vi "flash_RPCV3.vi"() -> ()   [LabVIEW 2017]
panel:
  in  "UDP Update":bool=TRUE
  out "error out 2":errorcluster
  out "Out 2":u8=2 format="%.0x"
  in  "Firmware":u16(ring)=2 items=["TDC"=4, "Middle"=3, "Backend"=2]
  out "Out":u8=1 format="%.0x"
  out "字符串 2":string
  out "concatenated string":string
  in  "Register_Base_Address":u32=512 format="%x"
  in  "start":bool=TRUE
  out "Current IP address":string="10.3.173.20"
  in  "IP address list":string[](array[string])=["10.3.173.20"]
  in  "回读":bool
  out "Current Progress":u32(slide)=6712320 scale=0.0..6712112.0
  out "error out":errorcluster={"status"=TRUE, "code"=1, "source"="TCP Close Connection in flash_RPCV3.vi"}
  out "appended array":bool[](array[boolean])
  out "Process":u32=6712320
  in  "error in (no error)":errorcluster
  in  "Read (TRUE)":bool
  out "byte data":string
  out "Total size (in bytes)":i64=6712112
  in  "bin file path (use dialog)":path=path "G:/rpc/aggregate/WR/firmware/NEM_DEVB/project_1.runs/impl_1/top.bin"
  # "FF80 0001 0000 0209 13"
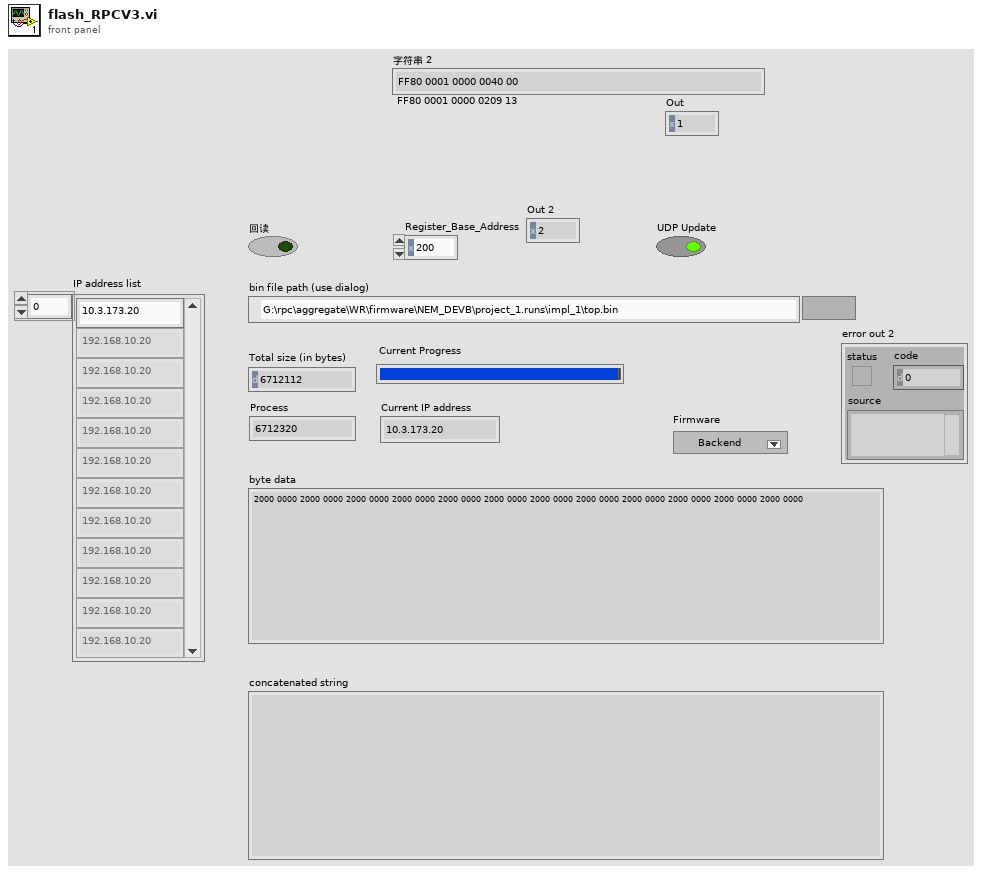
[diagram p1: front panel]
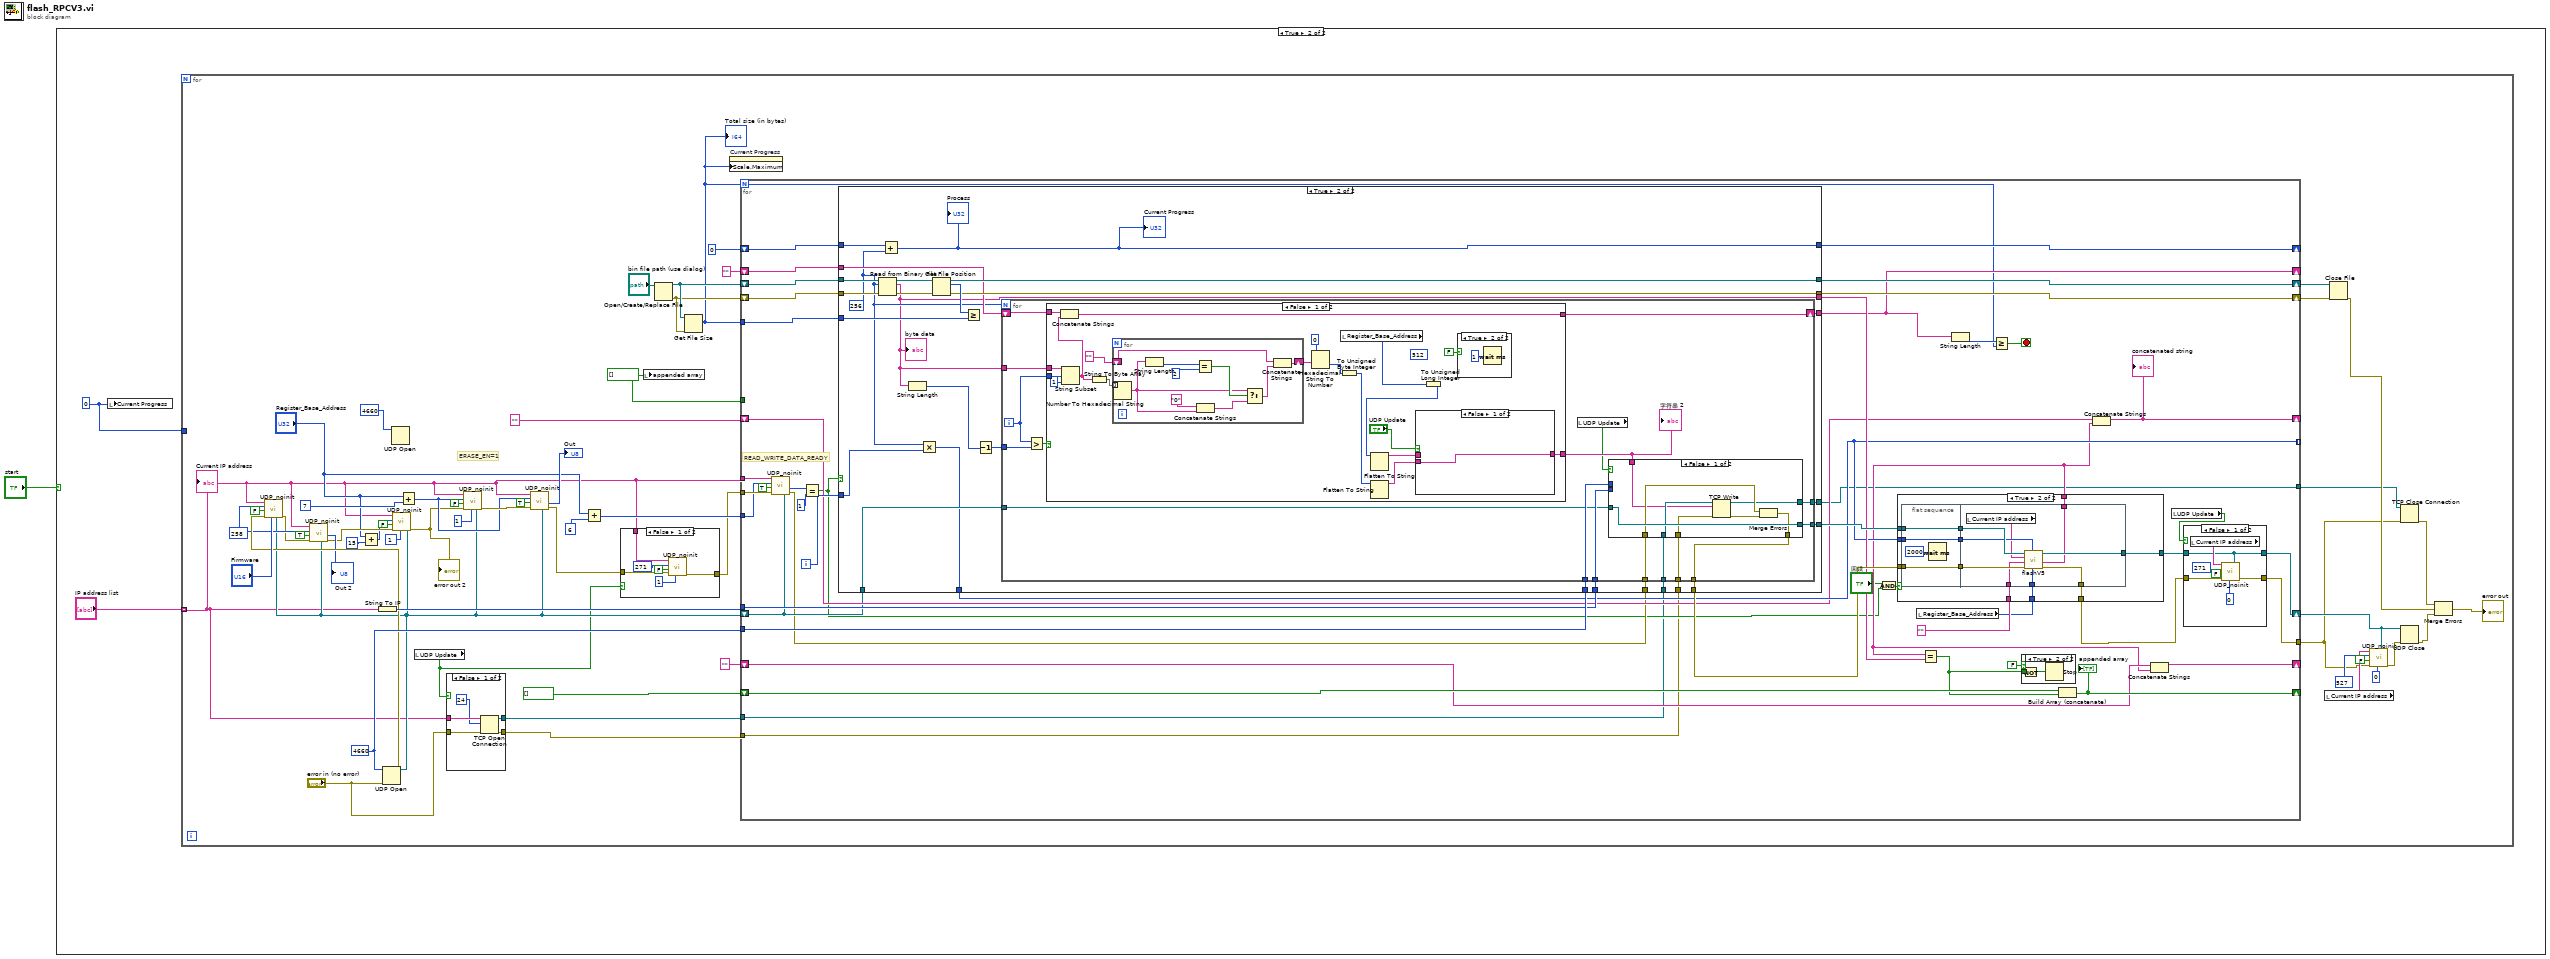
[diagram p0: block diagram]
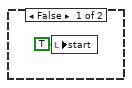
[diagram p2: hidden frame]
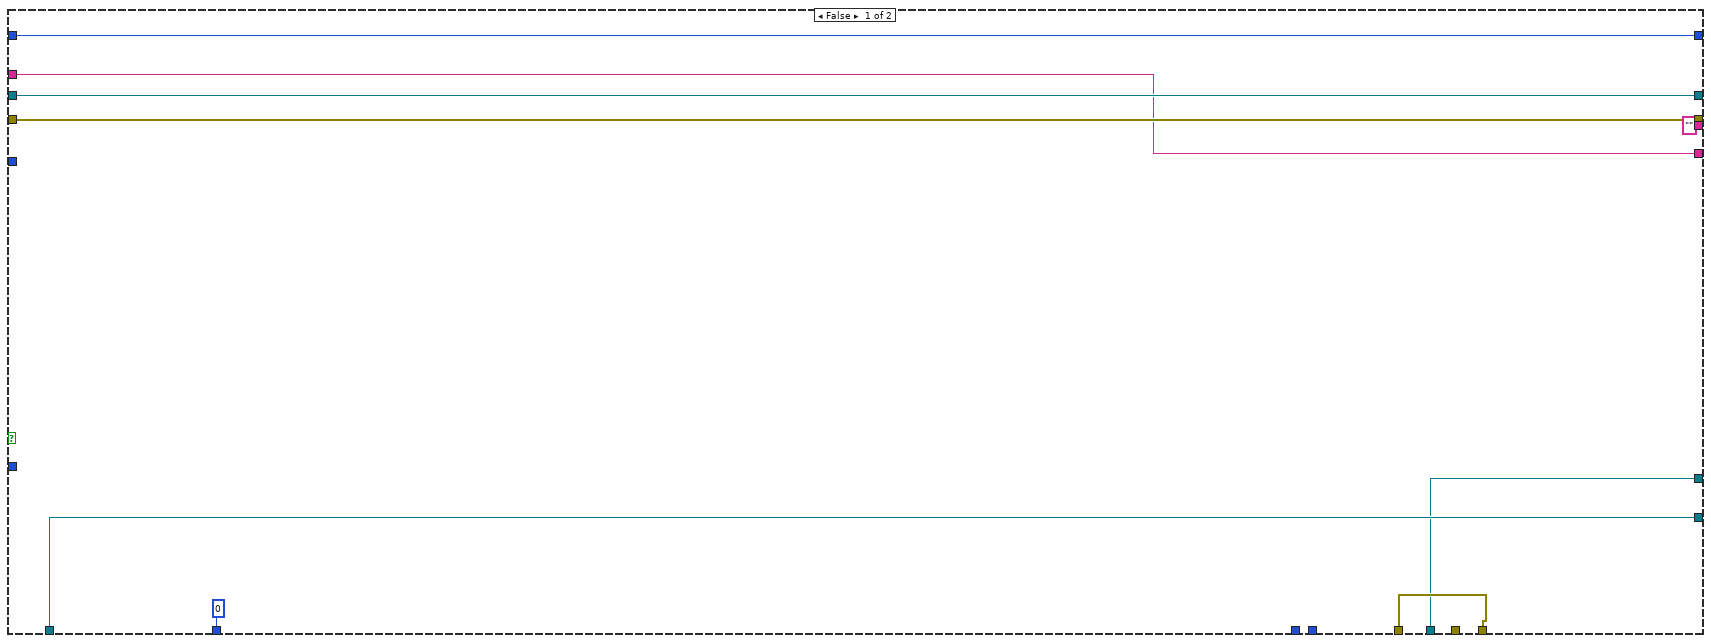
[diagram p6: hidden frame]
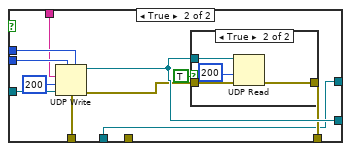
[diagram p7: hidden frame]
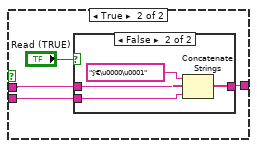
[diagram p9: hidden frame]
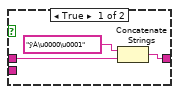
[diagram p10: hidden frame]
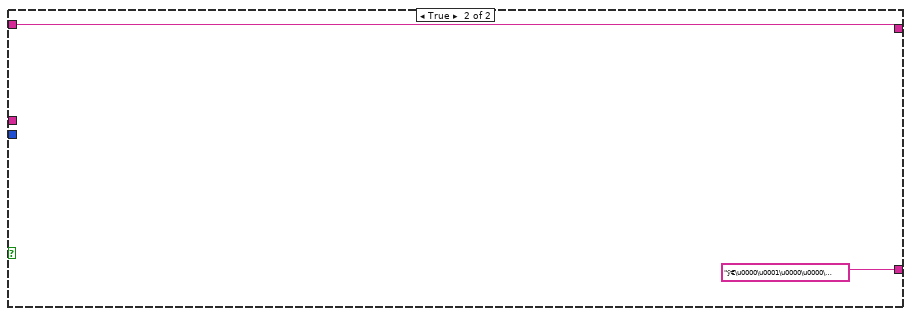
[diagram p12: hidden frame]
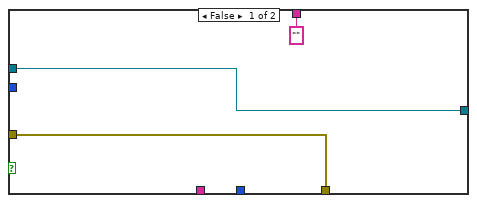
[diagram p13: hidden frame]
diagram:
  n1 = case shown="True" "start" {
    frame False {
      n2 = local write "start"(TRUE ("start")) -> ()
    }
    frame True {
      w3 = u8 0 ("In")
      n3 = local write "Current Progress"(w3) -> ()
      n4 = for {
        tunnel: "IP address list" -> [w6] mode=indexing
        tunnel: w3 -> [_]
        w33 = u32 258 ("Address")
        w46 = bool[] [] ("appended array")
        w57 = u16 4660 ("UDP port")
        # "ERASE_EN=1"
        n5 = Add(x="Register_Base_Address", y=u32 15 ("Address")) -> (x+y=w21:u32)
        n6 = String To IP(1:w6) -> (0:w56:u32)
        n7 = UDP Open(8:"error in (no error)", 11:w57) -> (port=w16:refnum<k16>, 0:w34:errorcluster)  [unwired: 3 in, 1 out]
        n8 = call "UDP_noinit.vi"("connection ID"=w16, "In"="Firmware", "error in (no error)"=w34, "Read (TRUE)"=FALSE, "Address"=w33, "IP address"=w6) -> ("error out"=w30:errorcluster)  [unwired: 2 in, 2 out]
        n9 = call "UDP_noinit.vi"("connection ID"=w16, "error in (no error)"=w30, "Read (TRUE)"=TRUE, "Address"=w33, "IP address"=w6) -> ("error out"=w23:errorcluster, "Out"=→"Out 2":u8)  [unwired: 3 in, 1 out]
        n10 = UDP Open(11:u16 4660 ("UDP port")) -> ()  [unwired: 4 in, 3 out]
        n11 = call "UDP_noinit.vi"("connection ID"=w16, "In"=u32 1 ("Address"), "error in (no error)"=w23, "Read (TRUE)"=FALSE, "Address"=w21, "IP address"=w6) -> ("error out"=w22:errorcluster)  [unwired: 2 in, 2 out]
        "error out 2" <- w22
        n12 = Add(x="Register_Base_Address", y=u32 7 ("Address")) -> (x+y=w41:u32)
        n13 = local read "UDP Update"() -> (w8:bool)
        n14 = case shown="False" w8 {
          tunnel: w6 -> [w74 _]
          tunnel: "error in (no error)" -> [w72 w75]
          tunnel: [w71 _] -> w13
          tunnel: [w70 w75] -> w12
          frame False {
            n15 = TCP Open Connection(address=w74, remote port or service name=u16 24 ("UDP port"), error in (no error)=w72) -> (connection ID=w71:refnum<k5>, error out=w70:errorcluster)  [unwired: 2 in]
          }
          frame True {
          }
        }
        n16 = call "UDP_noinit.vi"("connection ID"=w16, "In"=u8 1, "error in (no error)"=w22, "Read (TRUE)"=FALSE, "Address"=w41, "IP address"=w6) -> ("error out"=w50:errorcluster)  [unwired: 2 in, 2 out]
        n17 = call "UDP_noinit.vi"("connection ID"=w16, "error in (no error)"=w50, "Read (TRUE)"=TRUE, "Address"=w41, "IP address"=w6) -> ("error out"=w7:errorcluster, "Out"=→"Out":u8)  [unwired: 3 in, 1 out]
        n18 = Add(x="Register_Base_Address", y=u32 6 ("Address")) -> (x+y=w39:u32)
        n19 = case shown="False" w8 {
          tunnel: w7 -> [w68 w69]
          tunnel: w6 -> [w67 _]
          tunnel: [w64 w69] -> w5
          frame False {
            n20 = call "UDP_noinit.vi"("In"=u8 1, "error in (no error)"=w68, "Read (TRUE)"=FALSE, "Address"=u32 271, "IP address"=w67) -> ("error out"=w64:errorcluster)  [unwired: 3 in, 2 out]
          }
          frame True {
          }
        }
        n21 = local write "appended array"(w46) -> ()
        n22 = Open/Create/Replace File(file path (use dialog)="bin file path (use dialog)") -> (refnum out=w61:refnum<file>, error out=w60:errorcluster)  [unwired: 5 in, 1 out]
        n23 = Get File Size(file=w61, error in=w60) -> (size (in bytes)=w47:i64)  [unwired: 2 out]
        "Total size (in bytes)" <- w47
        n24 = property on="Current Progress" class="Slide (strict)"("Scale.Maximum"=w47) -> ()  [unwired: 2 in, 2 out]
        n25 = for {
          N: w47 -> [w103]
          tunnel: w47 -> [w122]
          shift-right: [w121] -> w59
          shift-left: w60 -> [w123]
          shift-right: [w120] -> w58
          shift-left: w61 -> [w124]
          shift-right: [w105] -> _
          shift-left: "" -> [w119]
          tunnel: w57 -> [w116]
          tunnel: [w77] -> w10
          tunnel: w56 -> [w115]
          shift-right: [w76] -> w25
          shift-left: w16 -> [w93]
          shift-right: [w117] -> _
          shift-left: u32 0 ("length (rest)") -> [w118]
          shift-right: [w110] -> _
          shift-left: bool[] [] -> [w108]
          tunnel: [w106] -> _ mode=indexing
          shift-right: [w101] -> _
          shift-left: "" -> [w100]
          tunnel: w6 -> [w98]
          tunnel: w5 -> [w92]
          shift-right: [w90] -> _
          shift-left: "" -> [w89]
          tunnel: w46 -> [_]
          tunnel: w39 -> [w85]
          tunnel: w13 -> [w83]
          tunnel: w12 -> [w82]
          tunnel: [w81] -> w11
          i -> [w111]
          stop <- w102 stop-if-true
          # "READ_WRITE_DATA_READY"
          n26 = call "UDP_noinit.vi"("connection ID"=w93, "error in (no error)"=w92, "Read (TRUE)"=TRUE, "Address"=w85, "IP address"=w98) -> ("error out"=w91:errorcluster, "Out"=w96:u8)  [unwired: 3 in, 1 out]
          n27 = Equal?(x=w96, y=u8 1) -> (x = y?=w87:bool)
          n28 = case shown="True" w87 {
            tunnel: w124 -> [w139 w169]
            tunnel: w123 -> [w140 w168]
            tunnel: w122 -> [_ w164]
            tunnel: [w140 w163] -> w121
            tunnel: [w139 w162] -> w120
            tunnel: w119 -> [w137 w161]
            tunnel: w118 -> [w138 w160]
            tunnel: [w138 w146] -> w117
            tunnel: w116 -> [_ w159]
            tunnel: w115 -> [_ w158]
            tunnel: w91 -> [w141 w157]
            tunnel: w93 -> [w142 w156]
            tunnel: [w142 w153] -> w114
            tunnel: [w141 w152] -> w113
            tunnel: w111 -> [_ w151]
            tunnel: ["" w149] -> w109
            tunnel: [0 w148] -> w106
            tunnel: [w137 w147] -> w105
            tunnel: w83 -> [w134 w145]
            tunnel: w82 -> [_ w144]
            tunnel: [w134 w143] -> w81
            frame False {
            }
            frame True {
              w150 = 256 ("count (1)")
              n29 = Read from Binary File(8:w168, 10:w150, 11:w169) -> (0:w166:errorcluster, 2:w149:string, 3:w167:refnum<file>)  [unwired: 3 in, 1 out]
              "byte data" <- w149
              n30 = Add(x=w160, y=w150) -> (x+y=w146:u32)
              "Process" <- w146
              "Current Progress" <- w146
              n31 = String Length(string=w149) -> (length=w155:i32)
              n32 = Multiply(x=w150, y=w151) -> (x*y=w148:i32)
              n33 = Get File Position(4:w166, 7:w167) -> (0:w163:errorcluster, 2:w165:i64, 3:w162:refnum<file>)
              n34 = Greater Or Equal?(x=w165, y=w164) -> ()  [unwired: 1 out]
              n35 = Decrement(x=w155) -> (x-1=w154:i32)
              n36 = for {
                N: w150 -> [_]
                tunnel: w149 -> [w186]
                shift-right: [w184] -> w147
                shift-left: w161 -> [w185]
                tunnel: w159 -> [w183]
                tunnel: w158 -> [w182]
                tunnel: w157 -> [w181]
                tunnel: w156 -> [w176]
                tunnel: [w174] -> w152
                tunnel: [w175] -> w153
                tunnel: w154 -> [w179]
                tunnel: w145 -> [w172]
                tunnel: w144 -> [w171]
                tunnel: [w170] -> w143
                i -> [w178]
                n37 = Greater?(x=w178, y=w179) -> (0:w180:bool)
                n38 = case shown="False" w180 {
                  tunnel: w186 -> [w222 _]
                  tunnel: w185 -> [w220 w253]
                  tunnel: [w219 w253] -> w184
                  tunnel: w178 -> [w214 _]
                  tunnel: [w213 "ÿ€\u0000\u0001\u0000\u0000\u0000@\u0000" ("字符串 2")] -> w177
                  frame False {
                    (unwired) u32 512 ("Address")
                    n39 = String Subset(string=w222, offset (0)=w214, length (rest)=1 ("length (rest)")) -> (substring=w218:string)
                    n40 = Concatenate Strings(w220, w218) -> (w219:string)
                    n41 = String To Byte Array(string=w218) -> (unsigned byte array=w228:u8[])
                    n42 = for {
                      shift-right: [w251] -> w227
                      shift-left: "" ("format string") -> [w248]
                      tunnel: w228 -> [w252] mode=indexing
                      n43 = Number To Hexadecimal String(2:w252) -> (0:w244:string)  [unwired: 1 in]
                      n44 = String Length(string=w244) -> (length=w250:i32)
                      n45 = Equal?(x=w250, y=2) -> (x = y?=w247:bool)
                      n46 = Concatenate Strings("0" ("format string"), w244) -> (w246:string)
                      n47 = Select(t=w244, s=w247, f=w246) -> (s? t:f=w243:string)
                      n48 = Concatenate Strings(w248, w243) -> (w251:string)
                    }
                    n49 = Hexadecimal String To Number(string=w227, default (0uL)=u64 0 ("default (0 U32)")) -> (number=w225:u64)  [unwired: 1 in, 1 out]
                    n50 = To Unsigned Byte Integer(number=w225) -> (unsigned 8bit integer=w224:u8)
                    n51 = local read "Register_Base_Address"() -> (w212:u32)
                    n52 = Flatten To String(anything=w224) -> (data string=w215:string)  [unwired: 3 in, 2 out]
                    n53 = To Unsigned Long Integer(number=w212) -> (unsigned 32bit integer=w223:u32)
                    n54 = Flatten To String(anything=w223) -> (data string=w216:string)  [unwired: 3 in, 2 out]
                    n55 = case shown="False" "UDP Update" {
                      tunnel: w216 -> [_ w234]
                      tunnel: w215 -> [w230 w233]
                      tunnel: [w230 w231] -> w213
                      frame False {
                      }
                      frame True {
                        n56 = case shown="False" "Read (TRUE)" {
                          tunnel: [w236 w240] -> w231
                          tunnel: w234 -> [w235 w239]
                          tunnel: w233 -> [_ w238]
                          frame True {
                            n57 = Concatenate Strings("ÿÀ\u0000\u0001" ("initial string"), w235) -> (w236:string)
                          }
                          frame False {
                            n58 = Concatenate Strings("ÿ€\u0000\u0001" ("initial string"), w239, w238) -> (w240:string)
                          }
                        }
                      }
                    }
                    n59 = case shown="True" FALSE {
                      frame False {
                      }
                      frame True {
                        n60 = Wait (ms)(milliseconds to wait=u32 1) -> ()  [unwired: 1 out]
                      }
                    }
                  }
                  frame True {
                  }
                }
                "字符串 2" <- w177
                n61 = local read "UDP Update"() -> (w173:bool)
                n62 = case shown="False" w173 {
                  tunnel: w183 -> [_ w205]
                  tunnel: w182 -> [_ w204]
                  tunnel: w181 -> [w191 w203]
                  tunnel: w177 -> [w188 w201]
                  tunnel: w176 -> [w194 w200]
                  tunnel: [w194 w199] -> w175
                  tunnel: [w189 w196] -> w174
                  tunnel: w172 -> [w193 w195]
                  tunnel: w171 -> [w192 _]
                  tunnel: [w187 w195] -> w170
                  frame False {
                    n63 = TCP Write(connection ID=w193, data in=w188, error in (no error)=w192) -> (connection ID out=w187:refnum<k5>, error out=w190:errorcluster)  [unwired: 1 in, 1 out]
                    n64 = Merge Errors(w191, w190) -> (w189:errorcluster)
                  }
                  frame True {
                    n65 = UDP Write(address=w204, port or service name=w205, connection ID=w200, data in=w201, 8:w203, 9:200 ("timeout ms (25000)")) -> (error out=w197:errorcluster, 3:w199:refnum<k16>)
                    n66 = case shown="True" TRUE {
                      tunnel: w199 -> [_ w210]
                      tunnel: w197 -> [w206 w209]
                      tunnel: [w206 w208] -> w196
                      frame False {
                      }
                      frame True {
                        n67 = UDP Read(connection ID=w210, timeout ms (25000)=200, 8:w209) -> (error out=w208:errorcluster)  [unwired: 5 out]
                      }
                    }
                  }
                }
              }
            }
          }
          n68 = And(x="回读", y=w87) -> (x .and. y?=w94:bool)
          n69 = local read "Register_Base_Address"() -> (w84:u32)
          n70 = case shown="True" w94 {
            tunnel: w114 -> [w257 w265]
            tunnel: [w257 w264] -> w80
            tunnel: w113 -> [w256 w263]
            tunnel: [w256 w262] -> w78
            tunnel: "" ("empty") -> [_ w261]
            tunnel: w106 -> [_ w260]
            tunnel: ["" ("String") w259] -> w88
            tunnel: w84 -> [_ w258]
            frame False {
            }
            frame True {
              n71 = flat-sequence {
                tunnel: w260 -> [w270]
                tunnel: w263 -> [w271]
                tunnel: w265 -> [w272]
                tunnel: [w272] -> w268
                tunnel: [w271] -> w267
                tunnel: [w270] -> w266
                tunnel: [w278] -> w262
                tunnel: w261 -> [w277]
                tunnel: [w276] -> w259
                tunnel: w268 -> [w281]
                tunnel: w267 -> [w279]
                tunnel: w266 -> [w275]
                tunnel: [w280] -> w264
                tunnel: w258 -> [w273]
                frame #0 {
                  n72 = Wait (ms)(milliseconds to wait=u32 2000) -> ()  [unwired: 1 out]
                }
                frame #1 {
                  n73 = local read "Current IP address"() -> (w274:string)
                  n74 = call "flashV5.vi"("Register_Base_Address"=w273, "flash_base_address"=w275, "error in (no error)"=w279, "empty"=w277, "address"=w274, "connection ID"=w281) -> ("error out"=w278:errorcluster, "String"=w276:string, "connection ID 2"=w280:refnum<k16>)  [unwired: 2 in, 1 out]
                }
              }
            }
          }
          n75 = Equal?(x=w88, y=w109) -> (x = y?=w107:bool)
          n76 = String Length(string=w105) -> (length=w104:i32)
          n77 = Greater Or Equal?(x=w104, y=w103) -> (x >= y?=w102:bool)
          n78 = case shown="True" FALSE {
            tunnel: w107 -> [_ w282]
            frame False {
            }
            frame True {
              n79 = Not(x=w282) -> (.not. x?=w283:bool)
              n80 = Stop(stop? (T)=w283) -> ()
            }
          }
          n81 = Build Array (concatenate)(w108, w107) -> (w110:bool[])
          "appended array" <- w110
          n82 = Concatenate Strings(w100, w88) -> (w101:string)
          "concatenated string" <- w101
          n83 = Concatenate Strings(w89, w88) -> (w90:string)
          n84 = local read "UDP Update"() -> (w79:bool)
          n85 = case shown="False" w79 {
            tunnel: w80 -> [w125 w132]
            tunnel: w78 -> [w131 w133]
            tunnel: [w130 w133] -> w77
            tunnel: [w125 w132] -> w76
            frame False {
              n86 = local read "Current IP address"() -> (w129:string)
              n87 = call "UDP_noinit.vi"("connection ID"=w125, "In"=u8 0, "error in (no error)"=w131, "Read (TRUE)"=FALSE, "Address"=u32 271, "IP address"=w129) -> ("error out"=w130:errorcluster)  [unwired: 2 in, 2 out]
            }
            frame True {
            }
          }
        }
        n88 = local read "Current IP address"() -> (w27:string)
        n89 = Close File(refnum=w58, error in=w59) -> (error out=w45:errorcluster)  [unwired: 1 out]
        n90 = call "UDP_noinit.vi"("connection ID"=w25, "In"=u8 0, "error in (no error)"=w10, "Read (TRUE)"=FALSE, "Address"=u32 527, "IP address"=w27) -> ("error out"=w26:errorcluster)  [unwired: 2 in, 2 out]
        n91 = UDP Close(connection ID=w25, 8:w26) -> (error out=w44:errorcluster)  [unwired: 1 out]
        n92 = TCP Close Connection(connection ID=w11, error in (no error)=w10) -> (error out=w9:errorcluster)  [unwired: 1 in, 1 out]
        n93 = Merge Errors(w9, w45, w44) -> (→"error out":errorcluster)
        "Current IP address" <- w6
      }
    }
  }
